vi "Agilent SNA Read Calibration Status.vi"(7 "Agilent SNA & SWP":T6, 8 "error in (no error)":errorcluster, 10 "Parameters to Measure":T2[](array[typedef]) {"Channel" min=1 max=99 step=1; "Parameter"."Stimulus Port" min=1 step=1; "Parameter"."Response Port" min=1 step=1}, 11 "VISA Resource Names":T7) -> (0 "error out":errorcluster {"code" format="%.0x"}, 1 "Parameters to Measure":T2[](array[typedef]) {"Channel" min=1 max=99 step=1; "Parameter"."Stimulus Port" min=1 step=1; "Parameter"."Response Port" min=1 step=1}, 2 "Calibration Type by Parameter":T1[](array[typedef]), 3 "dup VISA Resource Names":T7)   [LabVIEW 2011]
doc: "This VI for the HP 8753B is used to read the calibration type.\n\n0 response\n1 response and isolation\n2 S11 1-port\n3 S22 1-port\n4 full 2-port\n5 one path 2-port\n6 no cal detected"
uses:
  TypeDefs/Agilent SNA VISA.ctl
  TypeDefs/Agilent SNA Instrument Info.ctl
  tests/S Parameter/TypeDefs/SP Parameter to Measure.ctl
  tests/S Parameter/TypeDefs/SP Parameter.ctl
  tests/S Parameter/TypeDefs/SP Calibration State.ctl
  tests/S Parameter/TypeDefs/SP Measurement Format.ctl
  TypeDefs/Agilent SNA Calibration State.ctl
  TypeDefs/Agilent SNA Message Mode.ctl
  TypeDefs/Agilent SNA Measurement.ctl
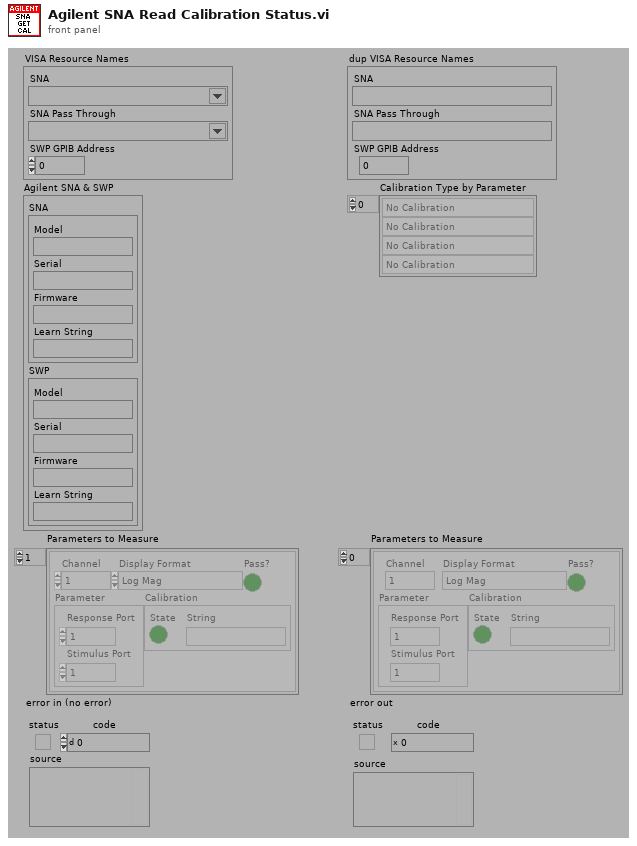
[diagram p1: front panel]
types:
  T1 = typedef "Agilent SNA Calibration State.ctl" = enum32{"No Calibration", "Calibrated"}
  T2 = typedef "SP Parameter to Measure.ctl" = cluster{"Channel":i8, "Parameter":T3, "Calibration":T4, "Display Format":T5, "Pass?":bool}
  T3 = typedef "SP Parameter.ctl" = cluster{"Stimulus Port":i8, "Response Port":i8}
  T4 = typedef "SP Calibration State.ctl" = cluster{"State":bool, "String":string}
  T5 = typedef "SP Measurement Format.ctl" = enum32{"Log Mag", "Phase", "Delay", "Smith (R+jX)", "Polar (Re/Im)", "Linear Mag", "SWR", "Real", "Imaginary", "Smith (Lin/Phase)", "Smith (Log/Phase)", "Smith (Real/Imag)", "Smith (G+jB)", "Polar (Lin/Phase)", "Polar (Log/Phase)", "Expanded Phase", "Positive Phase", "Inverted Smith", "Unwrapped Phase", "Power Out", "Power In", "Linear Mag/Phase", "Log Mag/Phase", "Real/Imaginary"}
  T6 = typedef "Agilent SNA Instrument Info.ctl" = cluster{"SNA":cluster{"Model":string, "Serial":string, "Firmware":string, "Learn String":string}, "SWP":cluster{"Model":string, "Serial":string, "Firmware":string, "Learn String":string}}
  T7 = typedef "Agilent SNA VISA.ctl" = cluster{"SNA":refnum<visa-resource-name>, "SNA Pass Through":refnum<visa-resource-name>, "SWP GPIB Address":i32}
  T8 = typedef "Agilent SNA Message Mode.ctl" = enum16{"On", "Off"}
  T9 = typedef "Agilent SNA Model.ctl" = enum16{"Not Supported", "8757X"}
  T10 = typedef "Agilent SNA Measurement.ctl" = enum32{"SXX", "A", "B", "C", "R", "A/B", "A/C", "A/R", "B/A", "B/C", "B/R", "C/A", "C/B", "C/R", "R/A", "R/B", "R/C", "Analog In - Aux In"}
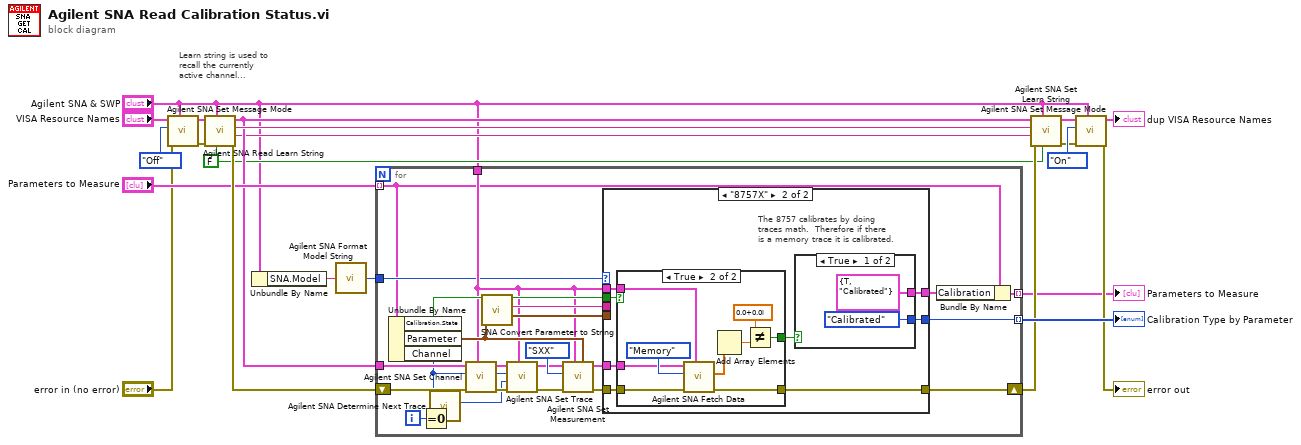
[diagram p0: block diagram]
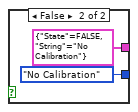
[diagram p4: hidden frame]
diagram:
  w13 = FALSE ("Get SWP Learn String? (T)")
  # "Learn string is used to\nrecall the currently \nactive channel..."
  n1 = call "Agilent SNA Set Message Mode.vi"("Agilent SNA & SWP"="Agilent SNA & SWP", "error in (no error)"="error in (no error)", "Message Mode"=Agilent_SNA_Message_Mode."Off", "VISA Resource Names"="VISA Resource Names") -> ("error out"=w4:errorcluster, "dup VISA Resource Names"=w3:T7)  [unwired: 6 out]
  n2 = call "Agilent SNA Read Learn String.vi"("Get SWP Learn String? (T)"=w13, "Agilent SNA & SWP"="Agilent SNA & SWP", "error in (no error)"=w4, "VISA Resource Names"=w3) -> ("error out"=w19:errorcluster, "SWP Learn String"=w14:string, "SNA Learn String"=w22:string, "dup VISA Resource Names"=w17:T7)  [unwired: 4 out]
  n3 = Unbundle By Name("Agilent SNA & SWP") -> ("SNA.Model"=w15:string)
  n4 = call "Agilent SNA Format Model String.vi"("Model String"=w15) -> ("Model"=w16:T9)
  n5 = for {
    tunnel: w17 -> [w42]
    shift-right: [w43] -> w20
    shift-left: w19 -> [w41]
    tunnel: "Parameters to Measure" -> [w25] mode=indexing
    tunnel: "Agilent SNA & SWP" -> [w33]
    tunnel: [w38] -> w21 mode=indexing
    tunnel: w16 -> [w26]
    tunnel: [w23] -> w1 mode=indexing
    i -> [w28]
    n6 = Unbundle By Name(w25) -> ("Calibration.State"=w40:bool, "Parameter"=w36:T3, "Channel"=w30:i8)
    n7 = Equal To 0?(x=w28) -> (x = 0?=w27:bool)
    n8 = call "Agilent SNA Determine Next Trace.vi"("Reset?"=w27, "Channel"=w30) -> ("Next Trace"=w29:i8)  [unwired: 9 out]
    n9 = call "Agilent SNA Set Channel.vi"("Agilent SNA & SWP"=w33, "error in (no error)"=w41, "Channel"=w30, "VISA Resource Names"=w42) -> ("error out"=w35:errorcluster, "dup VISA Resource Names"=w34:T7)  [unwired: 6 out]
    n10 = call "SNA Convert Parameter to String.vi"("Parameter"=w36) -> ("Parameter String"=w39:string)  [unwired: 10 out]
    n11 = call "Agilent SNA Set Trace.vi"("Agilent SNA & SWP"=w33, "error in (no error)"=w35, "Trace"=w29, "Channel"=w30, "VISA Resource Names"=w34) -> ("error out"=w31:errorcluster, "dup VISA Resource Names"=w32:T7)  [unwired: 5 out]
    n12 = call "Agilent SNA Set Measurement.vi"("Parameter"=w36, "Agilent SNA & SWP"=w33, "error in (no error)"=w31, "Measurement (SXX)"=Agilent_SNA_Measurement."SXX" ("Measurement (S11 - A/R)"), "VISA Resource Names"=w32) -> ("error out"=w45:errorcluster, "dup VISA Resource Names"=w44:T7)  [unwired: 3 in, 2 out]
    n13 = case shown="\"8757X\"" w26 {
      tunnel: w45 -> [w46 w52]
      tunnel: w44 -> [_ w53]
      tunnel: [w46 w51] -> w43
      tunnel: [_ w50] -> w38
      tunnel: w40 -> [_ w47]
      tunnel: w39 -> [_ _]
      tunnel: w33 -> [_ w54]
      tunnel: [_ w49] -> w24
      tunnel: w36 -> [_ _]
      frame "Not Supported" {
      }
      frame "8757X" {
        # "The 8757 calibrates by doing\ntraces math.  Therefore if there\nis a memory trace it is calibrated."
        n14 = case shown="True" w47 {
          tunnel: w54 -> [_ w64]
          tunnel: w53 -> [_ w61]
          tunnel: w52 -> [w55 w60]
          tunnel: [w55 w57] -> w51
          tunnel: [_ w56] -> w48
          frame False {
          }
          frame True {
            n15 = call "Agilent SNA Fetch Data.vi"("Agilent SNA & SWP"=w64, "error in (no error)"=w60, "Data to Read (Data)"=enum16{"Data", "Memory"}."Memory", "VISA Resource Names"=w61) -> ("error out"=w57:errorcluster, "Data (real+imag)"=w62:cdb[])  [unwired: 3 in, 3 out]
            n16 = Add Array Elements(numeric array=w62) -> (sum=w59:cdb)
            n17 = Not Equal?(x=cdb 0.0+0.0i, y=w59) -> (x != y?=w56:bool)
          }
        }
        n18 = case shown="True" w48 {
          tunnel: [Agilent_SNA_Calibration_State."Calibrated" ("S Parameter Test Cal Type") Agilent_SNA_Calibration_State."No Calibration" ("S Parameter Test Cal Type")] -> w50
          tunnel: [T4 {"State"=TRUE, "String"="Calibrated"} T4 {"State"=FALSE, "String"="No Calibration"}] -> w49
          frame True {
          }
          frame False {
          }
        }
      }
    }
    n19 = Bundle By Name(cluster=w25, "Calibration"=w24) -> (w23:T2)
  }
  "Parameters to Measure" <- w1
  "Calibration Type by Parameter" <- w21
  n20 = call "Agilent SNA Set Learn String.vi"("Set SWP Learn String? (T)"=w13, "Agilent SNA & SWP"="Agilent SNA & SWP", "error in (no error)"=w20, "SWP Learn String"=w14, "SNA Learn String"=w22, "VISA Resource Names"=w17) -> ("error out"=w9:errorcluster, "dup VISA Resource Names"=w10:T7)  [unwired: 1 in, 3 out]
  n21 = call "Agilent SNA Set Message Mode.vi"("Agilent SNA & SWP"="Agilent SNA & SWP", "error in (no error)"=w9, "Message Mode"=Agilent_SNA_Message_Mode."On", "VISA Resource Names"=w10) -> ("error out"=→"error out":errorcluster, "dup VISA Resource Names"=→"dup VISA Resource Names":T7)  [unwired: 6 out]
